vi "FAM Registers.vi"(0 "register instruction":T2) -> (4 "read completion":T1, 8 "IO Module\\Register Bus Idle":bool, 14 "ready for input":bool)   [LabVIEW 2015]
uses:
  <instrlib>/ni579x/Register Bus/v1/FPGA/Public/Register Instruction.ctl
  <instrlib>/ni579x/Register Bus/v1/FPGA/Public/Read Completion.ctl
  <instrlib>/ni579x/Config/v1/Shared/Types/ni579x Register Bus Subsystem ID.ctl
  <vilib>/rvi/eio/common/nirviEmuTemplateMethod_errors.vi
  <vilib>/eio/EIONode/EIONode.xnode
  <instrlib>/ni579x/Register Bus/v1/FPGA/ni579x Register Bus v1 FPGA.lvlib
  <vilib>/rvi/DataTransferAndStorage/Container/XNode/niFpgaContainer.xnode
  <vilib>/rvi/interface/RandomDataEmulation/nirviRandomDataFpgaReadWriteTemplate.vi
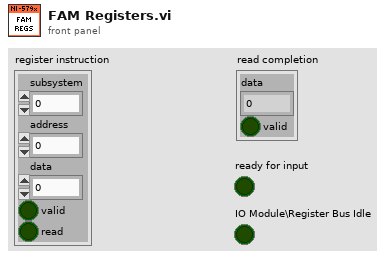
[diagram p1: front panel]
types:
  T1 = typedef "ni579x Register Bus v1 FPGA.lvlib/Read Completion.ctl" = cluster{"data":u32, "valid":bool}
  T2 = typedef "ni579x Register Bus v1 FPGA.lvlib/Register Instruction.ctl" = cluster{"subsystem":u8, "address":u16, "data":u32, "valid":bool, "read":bool}
  T3 = typedef "ni579x Register Bus Subsystem ID.ctl" = u8
  T4 = enum16{"Idle", "Loaded Address High", "Writing", "Reading"}
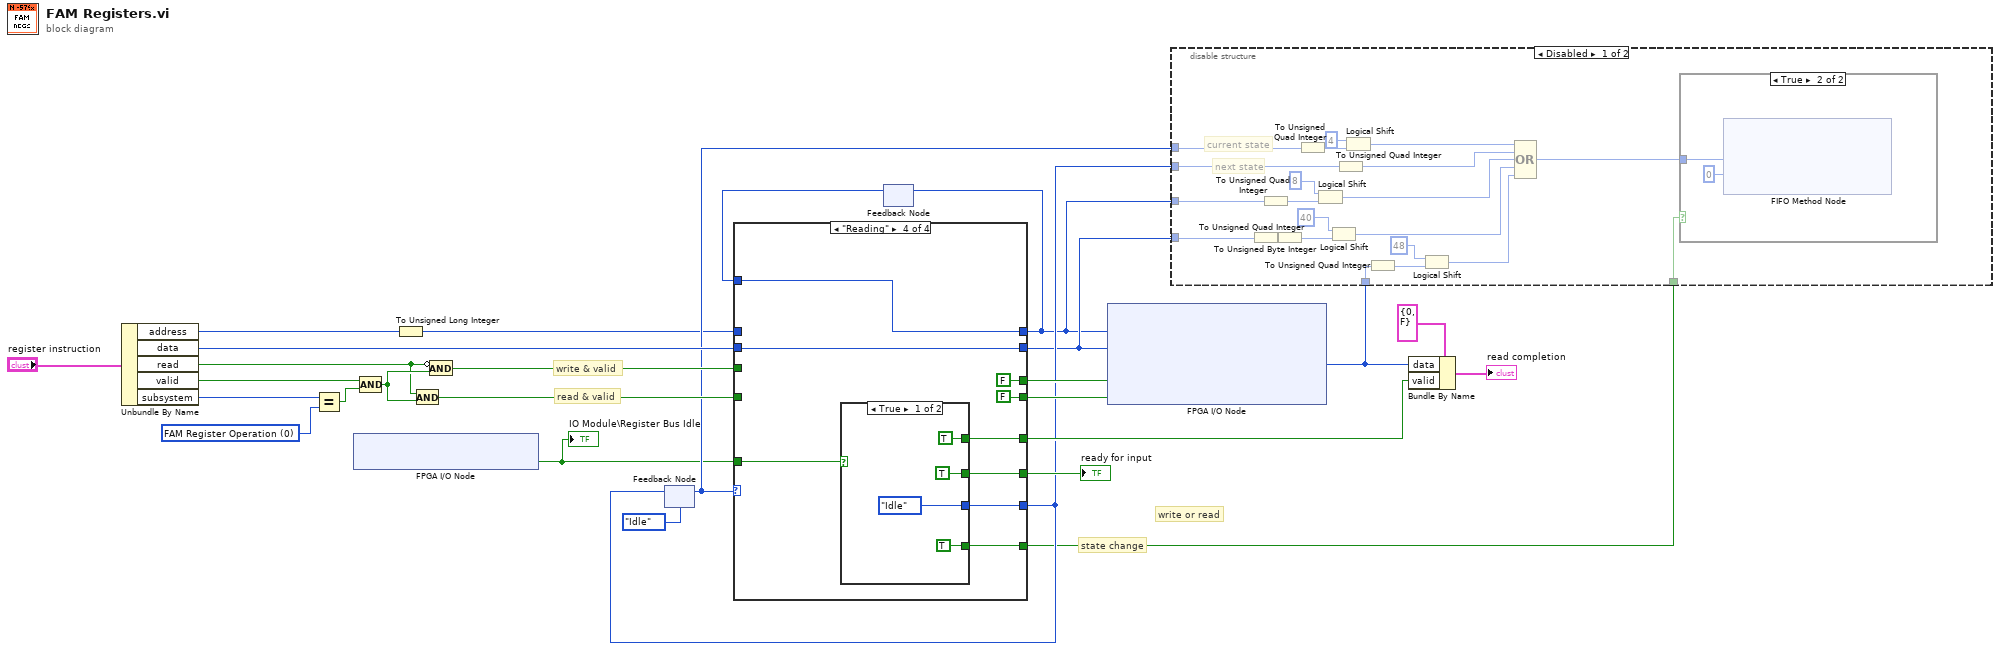
[diagram p0: block diagram]
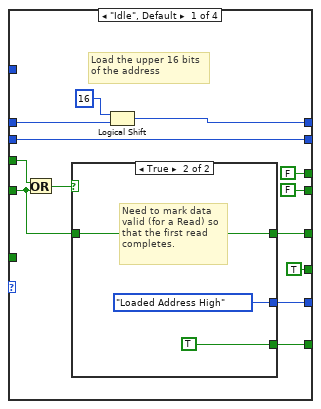
[diagram p4: hidden frame]
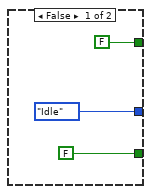
[diagram p5: hidden frame]
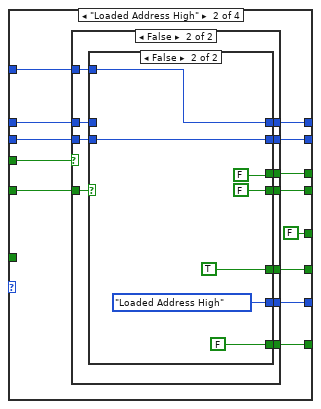
[diagram p6: hidden frame]
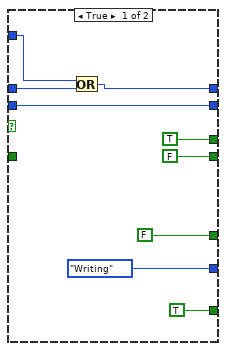
[diagram p7: hidden frame]
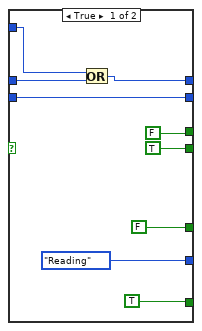
[diagram p8: hidden frame]
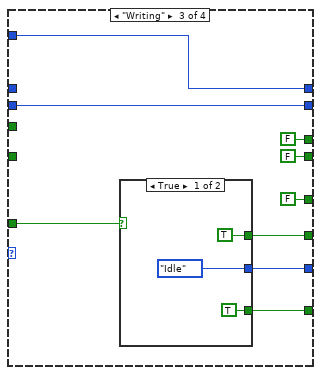
[diagram p9: hidden frame]
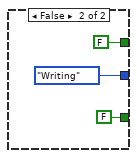
[diagram p10: hidden frame]
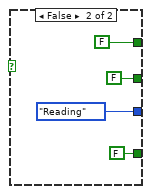
[diagram p11: hidden frame]
diagram:
  w2 = T3 0 items=["FAM Register Operation"=0, "User Command"=16, "Synchronization"=32] ("Subsystem ID")
  # "write or read"
  # "state change"
  # "read & valid"
  # "write & valid"
  n1 = Unbundle By Name("register instruction") -> ("address"=w23:u16, "data"=w22:u32, "read"=w25:bool, "valid"=w27:bool, "subsystem"=w1:u8)
  n2 = Equal?(x=w1, y=w2) -> (x = y?=w3:bool)
  n3 = xnode "FPGA I/O Node"() -> ("IO Module\\Register Bus Idle"=w4:bool)  [unwired: 1 in, 1 out]
  "IO Module\\Register Bus Idle" <- w4
  n4 = Compound Arithmetic op=AND(w27, w3) -> (w26:bool)
  n5 = To Unsigned Long Integer(number=w23) -> (unsigned 32bit integer=w5:u32)
  n6 = Compound Arithmetic op=AND(w25, w26) -> (w20:bool)
  n7 = Compound Arithmetic op=AND(invert w25, w26) -> (w21:bool)
  n8 = feedback #1(T4."Idle") -> (w12:T4)
  n9 = feedback #2() -> (w6:u32)  [unwired: 1 in]
  n10 = case shown="\"Reading\"" w12 {
    tunnel: w5 -> [w39 w47 _ _]
    tunnel: w22 -> [w38 w49 w102 w117]
    tunnel: w21 -> [w37 w59 _ _]
    tunnel: w20 -> [w28 w56 _ _]
    tunnel: [w30 w50 w96 w111] -> w7
    tunnel: [w38 w48 w102 w117] -> w10
    tunnel: [FALSE w58 FALSE FALSE] -> w18
    tunnel: [FALSE w57 FALSE FALSE] -> w19
    tunnel: [w35 w55 w99 w115] -> w11
    tunnel: [w29 FALSE FALSE w113] -> w13
    tunnel: w4 -> [_ _ w100 w116]
    tunnel: [TRUE w54 w98 w114] -> w16
    tunnel: [w34 w52 w97 w112] -> w8
    tunnel: w6 -> [_ w51 w96 w111]
    frame "Idle", Default {
      # "Load the upper 16 bits\nof the address"
      n11 = Or(x=w37, y=w28) -> (x .or. y?=w36:bool)
      n12 = case shown="True" w36 {
        tunnel: [T4."Idle" T4."Loaded Address High"] -> w35
        tunnel: [FALSE TRUE] -> w34
        tunnel: [FALSE w44] -> w29
        tunnel: w28 -> [_ w44]
        frame False {
        }
        frame True {
          # "Need to mark data \nvalid (for a Read) so\nthat the first read \ncompletes."
        }
      }
      n13 = Logical Shift(y=i16 16, x=w39) -> (x << y=w30:u32)
    }
    frame "Loaded Address High" {
      n14 = case shown="False" w59 {
        tunnel: [FALSE w79] -> w58
        tunnel: [TRUE w78] -> w57
        tunnel: w56 -> [_ w77]
        tunnel: [T4."Writing" w76] -> w55
        tunnel: [FALSE w75] -> w54
        tunnel: [TRUE w74] -> w52
        tunnel: w51 -> [w61 w73]
        tunnel: [w60 w72] -> w50
        tunnel: w49 -> [w63 w71]
        tunnel: [w63 w70] -> w48
        tunnel: w47 -> [w62 w69]
        frame True {
          n15 = Or(x=w61, y=w62) -> (x .or. y?=w60:u32)
        }
        frame False {
          n16 = case shown="False" w77 {
            tunnel: [TRUE FALSE] -> w79
            tunnel: [FALSE FALSE] -> w78
            tunnel: [T4."Reading" T4."Loaded Address High"] -> w76
            tunnel: [FALSE TRUE] -> w75
            tunnel: [TRUE FALSE] -> w74
            tunnel: w73 -> [w82 w90]
            tunnel: [w80 w90] -> w72
            tunnel: [w83 w89] -> w70
            tunnel: w71 -> [w83 w89]
            tunnel: w69 -> [w81 _]
            frame True {
              n17 = Or(x=w82, y=w81) -> (x .or. y?=w80:u32)
            }
            frame False {
            }
          }
        }
      }
    }
    frame "Writing" {
      n18 = case shown="True" w100 {
        tunnel: [T4."Idle" T4."Writing"] -> w99
        tunnel: [TRUE FALSE] -> w98
        tunnel: [TRUE FALSE] -> w97
        frame True {
        }
        frame False {
        }
      }
    }
    frame "Reading" {
      n19 = case shown="True" w116 {
        tunnel: [T4."Idle" T4."Reading"] -> w115
        tunnel: [TRUE FALSE] -> w114
        tunnel: [TRUE FALSE] -> w113
        tunnel: [TRUE FALSE] -> w112
        frame True {
        }
        frame False {
        }
      }
    }
  }
  "ready for input" <- w16
  n20 = feedback-in #1(w11) -> ()
  n21 = feedback-in #2(w7) -> ()
  n22 = xnode "FPGA I/O Node"("IO Module\\Register Bus Address"=w7, "IO Module\\Register Bus Write Data"=w10, "IO Module\\Register Bus Write"=w19, "IO Module\\Register Bus Read"=w18) -> ("IO Module\\Register Bus Read Data"=w9:u16)  [unwired: 5 in, 5 out]
  n23 = disable-structure shown="Disabled" {
    disable-tunnel: w12 -> [w148 _]
    disable-tunnel: w11 -> [w145 _]
    disable-tunnel: w7 -> [w143 _]
    disable-tunnel: w10 -> [w139 _]
    disable-tunnel: w9 -> [w135 _]
    disable-tunnel: w8 -> [w128 _]
    frame Disabled {
      # "next state"
      # "current state"
      n24 = To Unsigned Byte Integer(number=w139) -> (unsigned 8bit integer=w138:u8)
      n25 = To Unsigned Quad Integer(1:w143) -> (0:w142:u64)
      n26 = To Unsigned Quad Integer(1:w138) -> (0:w141:u64)
      n27 = To Unsigned Quad Integer(1:w148) -> (0:w147:u64)
      n28 = Logical Shift(y=i8 8, x=w142) -> (x << y=w132:u64)
      n29 = Logical Shift(y=i8 40, x=w141) -> (x << y=w131:u64)
      n30 = To Unsigned Quad Integer(1:w145) -> (0:w133:u64)
      n31 = Logical Shift(y=i8 4, x=w147) -> (x << y=w134:u64)
      n32 = To Unsigned Quad Integer(1:w135) -> (0:w137:u64)
      n33 = Logical Shift(y=i8 48, x=w137) -> (x << y=w130:u64)
      n34 = Compound Arithmetic op=OR(w134, w133, w132, w131, w130) -> (w129:u64)
      n35 = case shown="True" w128 {
        tunnel: w129 -> [_ w150]
        frame False {
        }
        frame True {
          n36 = xnode ("FIFO Method Node")("Element"=w150, "Timeout"=0) -> ()  [unwired: 1 in, 2 out]
        }
      }
    }
    frame Enabled {
    }
  }
  n37 = Bundle By Name(cluster=T1 {"data"=0, "valid"=FALSE} ("read completion"), "data"=w9, "valid"=w13) -> (→"read completion":T1)
